vi "validate_paths.vi"(8 "error in (no error)":errorcluster, 10 "File or Directory input":path, 11 "Target zip file input":path) -> (0 "error out":errorcluster, 1 "Invalid Path?":bool, 2 "File or Directory selected":path, 3 "Target zip file selected":path)   [LabVIEW 2010, in "ErrorController.lvclass"]
uses:
  ErrorController.lvclass
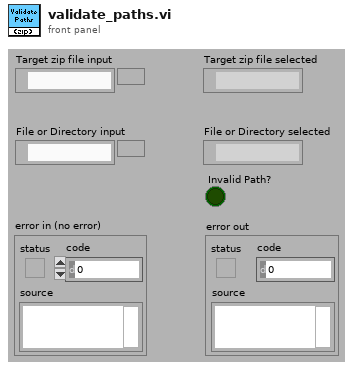
[diagram p1: front panel]
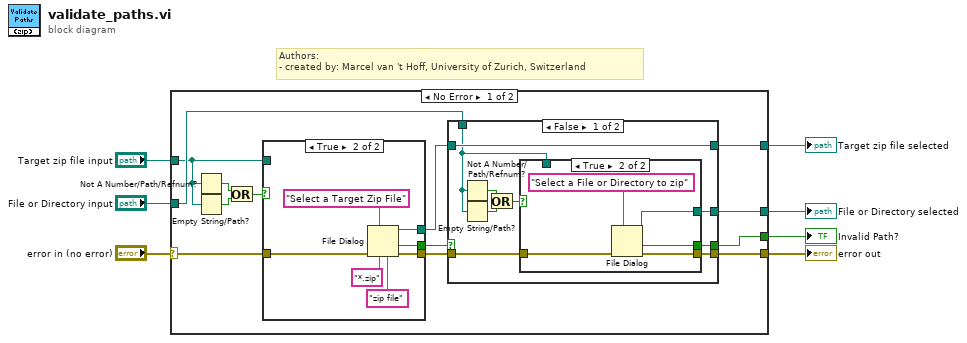
[diagram p0: block diagram]
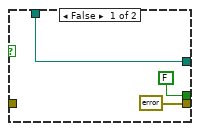
[diagram p2: hidden frame]
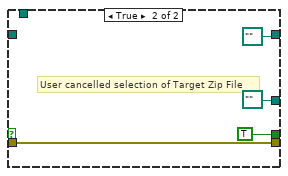
[diagram p3: hidden frame]
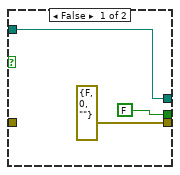
[diagram p4: hidden frame]
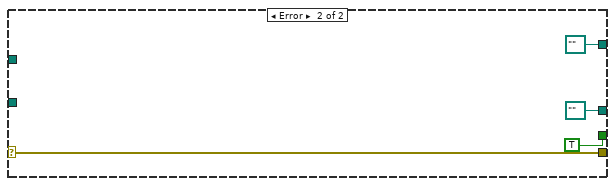
[diagram p5: hidden frame]
diagram:
  # "Authors: \n- created by: Marcel van 't Hoff, University of Zurich, Switzerland"
  n1 = case shown="No Error" "error in (no error)" {
    selector: "error in (no error)" -> [w10 w55]
    tunnel: [w16 w55] -> w7
    tunnel: "Target zip file input" -> [w9 _]
    tunnel: "File or Directory input" -> [w12 _]
    tunnel: [w11 TRUE ("cancelled")] -> w3
    tunnel: [w13 path "" ("File or Directory input")] -> w2
    tunnel: [w14 path ""] -> w1
    frame No Error {
      n2 = Not A Number/Path/Refnum?(number/path/refnum=w9) -> (NaN/Path/Refnum?=w19:bool)
      n3 = Empty String/Path?(string/path=w9) -> (empty?=w20:bool)
      n4 = Or(x=w19, y=w20) -> (x .or. y?=w8:bool)
      n5 = case shown="True" w8 {
        tunnel: [FALSE ("cancelled") w50] -> w17
        tunnel: [errorcluster {"status"=FALSE, "code"=0, "source"=""} ("error out") w49] -> w18
        tunnel: w9 -> [w42 _]
        tunnel: [w42 w48] -> w15
        tunnel: w10 -> [_ w47]
        frame False {
        }
        frame True {
          n6 = File Dialog(4:"zip file" ("pattern label"), 6:"*.zip" ("pattern (all files)"), 7:"Select a Target Zip File" ("prompt"), 8:w47) -> (0:w49:errorcluster, 1:w50:bool, 3:w48:path)  [unwired: 4 out]
        }
      }
      n7 = case shown="False" w17 {
        tunnel: w18 -> [w26 w39]
        tunnel: [w25 w39] -> w16
        tunnel: w15 -> [w24 _]
        tunnel: [w24 path "" ("File or Directory input")] -> w14
        tunnel: [w23 path "" ("Target zip file input")] -> w13
        tunnel: w12 -> [w22 _]
        tunnel: [w21 TRUE ("cancelled")] -> w11
        frame False {
          n8 = Not A Number/Path/Refnum?(number/path/refnum=w22) -> (NaN/Path/Refnum?=w28:bool)
          n9 = Empty String/Path?(string/path=w22) -> (empty?=w27:bool)
          n10 = Or(x=w28, y=w27) -> (x .or. y?=w29:bool)
          n11 = case shown="True" w29 {
            tunnel: [w30 w37] -> w23
            tunnel: [FALSE ("cancelled") w35] -> w21
            tunnel: [errorcluster {"status"=FALSE, "code"=0, "source"=""} ("error out") w34] -> w25
            tunnel: w26 -> [_ w33]
            tunnel: w22 -> [w30 _]
            frame False {
            }
            frame True {
              n12 = File Dialog(7:"Select a File or Directory to zip" ("prompt"), 8:w33) -> (0:w34:errorcluster, 1:w35:bool, 3:w37:path)  [unwired: 6 out]
            }
          }
        }
        frame True {
          # "User cancelled selection of Target Zip File"
        }
      }
    }
    frame Error {
    }
  }
  "error out" <- w7
  "Target zip file selected" <- w1
  "File or Directory selected" <- w2
  "Invalid Path?" <- w3
